vi "TempControl.vi"() -> ()   [LabVIEW 2020]
doc: "This VI is a solution to an exercise in the LabVIEW Basics I course.\n\nThis VI acquires temperature values every 500 ms and also takes a running average of the last three temperature measurements and displays both the raw data and the running average in the strip chart."
panel:
  out "Warning":bool
  in  "high limit":dbl
  out "Temperature History":cluster{dbl, "Temperature":dbl}(graph)
  in  "Power":bool=TRUE
  # "ON\n\nOFF"
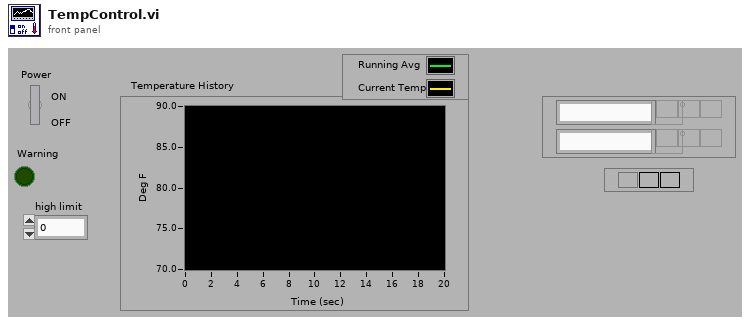
[diagram p1: front panel]
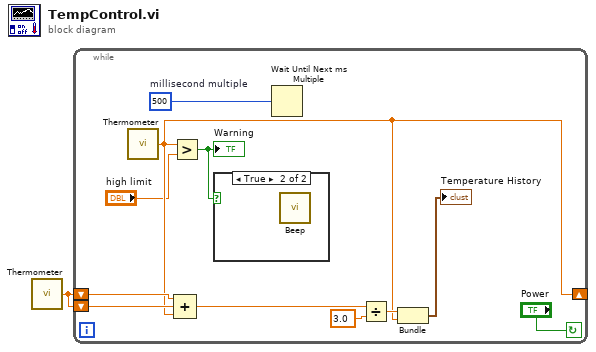
[diagram p0: block diagram]
diagram:
  n1 = call "Thermometer.vi"() -> ("Temperature"=w1:dbl)  [unwired: 1 in]
  n2 = while {
    shift-left: w1 -> [w8]
    shift-left: w1 -> [w9]
    shift-right: [w4] -> _
    stop <- "Power" continue-if-true
    w11 = u32 500  # millisecond multiple
    n3 = call "Thermometer.vi"() -> ("Temperature"=w4:dbl)  [unwired: 1 in]
    n4 = Greater?(x=w4, y="high limit") -> (0:w2:bool)
    "Warning" <- w2
    n5 = Compound Arithmetic op=ADD(w9, w8, w4) -> (w7:dbl)
    n6 = case shown="True" w2 {
      frame False {
      }
      frame True {
        n7 = call <vilib>:"Beep.vi"() -> ()  [unwired: 12 in]
      }
    }
    n8 = Wait Until Next ms Multiple(millisecond multiple=w11) -> ()  [unwired: 1 out]
    n9 = Divide(x=w7, y=3.0 ("number: 0 to 1")) -> (x/y=w6:dbl)
    n10 = Bundle(w6, "Temperature"=w4) -> (→"Temperature History":cluster{dbl, "Temperature":dbl})  [unwired: 1 in]
  }
